vi "PID.vi"(0 "array":waveform(dbl)[](array[waveform])=[{"t0"=timestamp(3657553104.2081175 s since 1904-01-01), "dt"=9.999999999999999e-05, "Y"=array[10780 elements], "attributes"=variant("NI_ChannelName"=variant(string "Mic Ref"), "NI_UnitDescription"=variant(string "Volts"))}, {"t0"=timestamp(3657553104.2081285 s since 1904-01-01), "dt"=9.999999999999999e-05, "Y"=array[10780 elements], "attributes"=variant("NI_ChannelName"=variant(string "Mic Active"), "NI_UnitDescription"=variant(string "Volts"))}, {"t0"=timestamp(3657553104.2081394 s since 1904-01-01), "dt"=9.999999999999999e-05, "Y"=array[10780 elements], "attributes"=variant("NI_ChannelName"=variant(string "Heater Voltage"), "NI_UnitDescription"=variant(string "Volts"))}, {"t0"=timestamp(3657553104.2081504 s since 1904-01-01), "dt"=9.999999999999999e-05, "Y"=array[10780 elements], "attributes"=variant("NI_ChannelName"=variant(string "Heater Shunt"), "NI_UnitDescription"=variant(string "Volts"))}, {"t0"=timestamp(3657553104.2081614 s since 1904-01-01), "dt"=9.999999999999999e-05, "Y"=array[10780 elements], "attributes"=variant("NI_ChannelName"=variant(string "Diode Voltage"), "NI_UnitDescription"=variant(string "Volts"))}], 1 "output range":cluster{"output high":dbl, "output low":dbl}={"output high"=2.0, "output low"=0.0}, 2 "Bandwidth":i32=1 format="%.1f", 3 "autotuning parameters":T1={"technique"=1, "type of controller"=1, "control specification"=0, "amplitude"=0.5} {"amplitude" format="%.2f"; "control specification" items=["normal", "fast", "slow"]; "type of controller" items=["P", "PI", "PID"]; "technique" items=["Step Open Loop", "Step Closed Loop", "Relay", "PID Relay"]}, 5 "index":i32=4, 6 "Setpoint":dbl=52.5, 7 "manual control":dbl=1.6, 9 "Frequency":i32=70, 10 "reinitialize? (F)":bool, 11 "error in (no error)":errorcluster, 12 "auto? (F)":bool=TRUE, 13 "PID gains":T2={"proportional gain (Kc)"=0.0125, "integral time (Ti, min)"=2.0, "derivative time (Td, min)"=0.0} {"derivative time (Td, min)" format="%.3f"; "integral time (Ti, min)" format="%.3f"; "proportional gain (Kc)" format="%.3f"}) -> (4 "output":dbl=1.578036883905017 format="%.2f", 8 "Channel name":string="Diode Voltage", 14 "Input":dbl=52.51542673351115, 15 "error out":errorcluster)   [LabVIEW 2019]
doc: "This example demonstrates how to acquire a continuous amount of data (Waveform) using the DAQ device's internal clock. It also shows how to synchronize two devices for different device families (E Series, S Series, M Series, X Series, DSA, and SC Express), to simultaneously acquire the data.\n\nFor instructions on how to connect your signals to the DAQ device, refer to your device documentation."
uses:
  <vilib>/addons/control/pid/autopid.llb/PID autotuning parameters (adv).ctl
  <vilib>/Waveform/WDTOps.llb/WDT Get Final Time Value DBL.vi
  <vilib>/addons/control/pid/NI_PID_autopid.lvlib
  <vilib>/Analysis/NI_AALPro.lvlib
panel:
  # "PID"
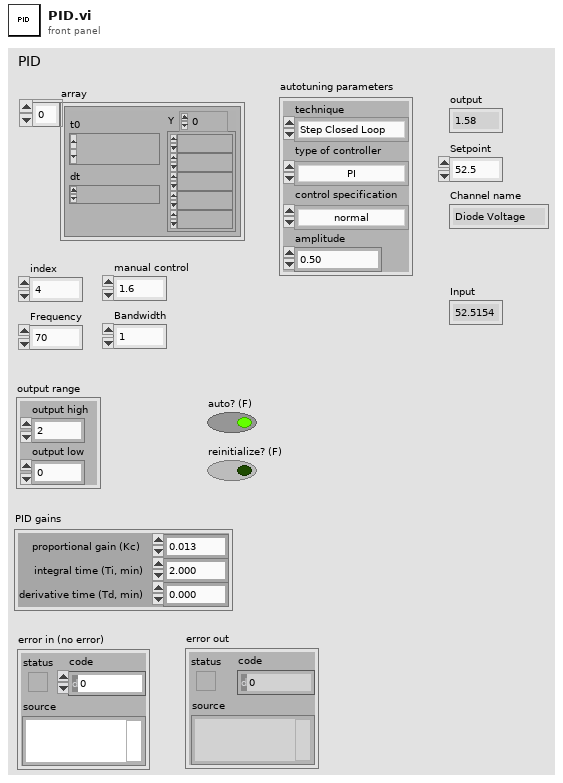
[diagram p1: front panel]
types:
  T1 = typedef "NI_PID_autopid.lvlib/PID autotuning parameters (adv).ctl" = cluster{"technique":u16, "type of controller":u16, "control specification":u16, "amplitude":dbl}
  T2 = cluster{"proportional gain (Kc)":dbl, "integral time (Ti, min)":dbl, "derivative time (Td, min)":dbl}
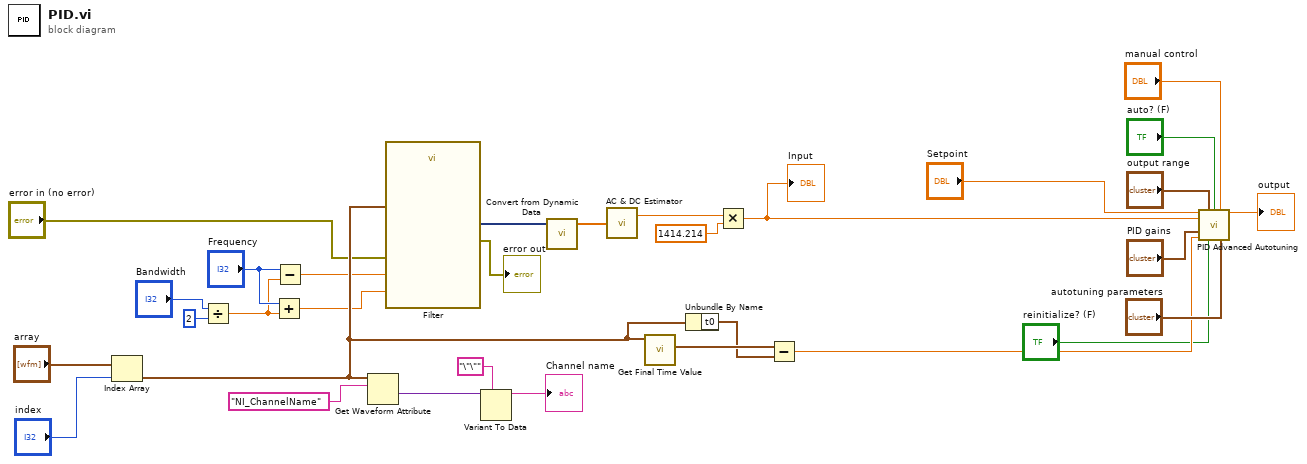
[diagram p0: block diagram]
diagram:
  n1 = Index Array(array="array", index="index") -> (element=w21:waveform(dbl))
  n2 = Divide(x="Bandwidth", y=2) -> (x/y=w16:dbl)
  n3 = Add(x="Frequency", y=w16) -> (x+y=w14:dbl)
  n4 = Subtract(x="Frequency", y=w16) -> (x-y=w15:dbl)
  n5 = Get Waveform Attribute(6:"NI_ChannelName" ("name"), 7:w21) -> (1:w22:variant)  [unwired: 2 in, 3 out]
  n6 = call "Filter"("error in (no error)"="error in (no error)", "Lower Cut-Off"=w15, "Upper Cut-Off"=w14, "Signal"=w21) -> ("error out"=→"error out":errorcluster, "Filtered Signal"=w13:dynamicdata)  [unwired: 6 in]
  n7 = Variant To Data(type="\"\"" ("name"), Variant=w22) -> (data=→"Channel name":string)  [unwired: 1 in, 1 out]
  n8 = call "Convert from Dynamic Data"("Dynamic Data Type"=w13) -> ("Array"=w12:dbl[])  [unwired: 3 in]
  n9 = call <vilib>:"AC & DC Estimator.vi"("Signal (V)"=w12) -> ("AC estimate (Vrms)"=w10:dbl)  [unwired: 1 out]
  n10 = call-poly <vilib>:"Get Final Time Value.vi"("waveform in"=w21) -> ("tf"=w26:timestamp)  [unwired: 8 in, 2 out]
  n11 = Unbundle By Name(w21) -> ("t0"=w25:timestamp)
  n12 = Multiply(x=w10, y=1414.214) -> (x*y=w5:dbl)
  "Input" <- w5
  n13 = Subtract(x=w26, y=w25) -> (x-y=w6:dbl)
  n14 = call <vilib>:"PID Advanced Autotuning.vi"("setpoint"="Setpoint", "output range"="output range", "auto? (F)"="auto? (F)", "manual control"="manual control", "process variable"=w5, "PID gains"="PID gains", "dt (s)"=w6, "reinitialize? (F)"="reinitialize? (F)", "autotuning parameters"="autotuning parameters") -> ("output"=→"output":dbl)  [unwired: 4 in, 2 out]
